vi "doAction.vi"(8 "error in (no error)":errorcluster, 11 "Run in":refnum<class "Run.lvclass">) -> (0 "error out":errorcluster, 3 "Run out":refnum<class "Run.lvclass">)   [LabVIEW 2018, in "Run.lvclass"]
uses:
  Run.lvclass
  State/State.lvclass
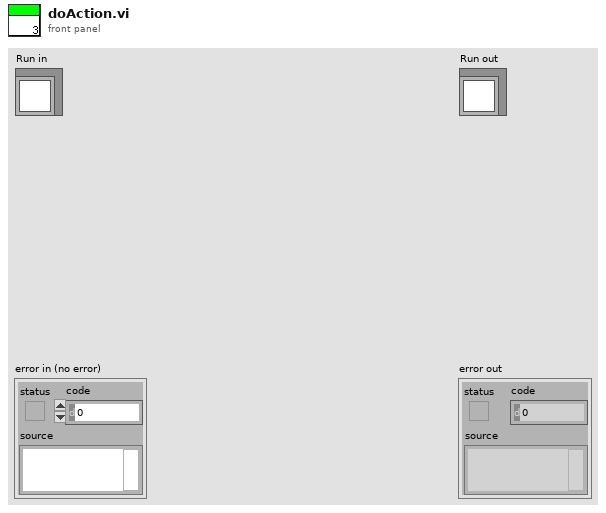
[diagram p1: front panel]
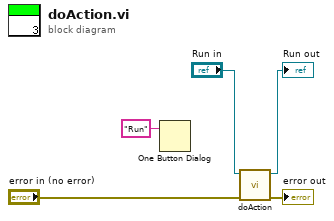
[diagram p0: block diagram]
diagram:
  n1 = One Button Dialog(message="Run") -> ()  [unwired: 1 in, 1 out]
  n2 = call-parent "doAction.vi"("error in (no error)"="error in (no error)", "State in"="Run in") -> ("error out"=→"error out":errorcluster, "State out"=→"Run out":refnum<class "Run.lvclass">)  [unwired: 8 in]
